vi "删除字母.vi"(10 "输入字符串":string) -> (2 "输出字符串":string)   [LabVIEW 2016]
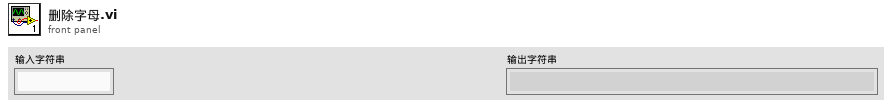
[diagram p1: front panel]
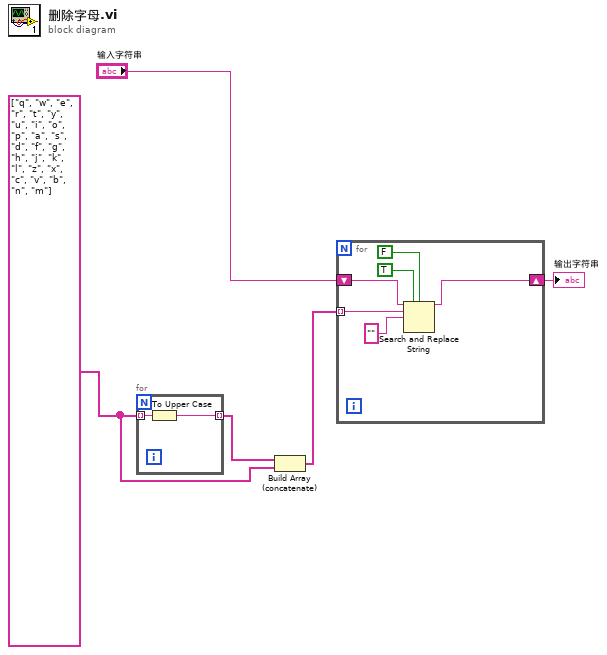
[diagram p0: block diagram]
diagram:
  w4 = string[] ["q", "w", "e", "r", "t", "y", "u", "i", "o", "p", "a", "s", "d", "f", "g", "h", "j", "k", "l", "z", "x", "c", "v", "b", "n", "m"]
  n1 = for {
    tunnel: w4 -> [w7] mode=indexing
    tunnel: [w6] -> w3 mode=indexing
    n2 = To Upper Case(1:w7) -> (0:w6:string)
  }
  n3 = Build Array (concatenate)(w3, w4) -> (w2:string[])
  n4 = for {
    tunnel: w2 -> [w13] mode=indexing
    shift-right: [w10] -> w5
    shift-left: "输入字符串" -> [w11]
    n5 = Search and Replace String(replace all?=TRUE ("replace all? (F)"), case sensitive?=FALSE ("ignore case? (F)"), input string=w11, search string=w13, replace string="") -> (result string=w10:string)  [unwired: 3 in, 3 out]
  }
  "输出字符串" <- w5
